vi "SubVI-AOMvolt-Power Calibration for 1064-v3.vi"() -> ()   [LabVIEW 2014]
uses:
  <vilib>/DAQmx/read.llb/DAQmx Read (Analog 1D DBL 1Chan NSamp).vi
  <vilib>/Analysis/NI_AALBase.lvlib
  <vilib>/Analysis/baseanly.llb/Mean (DBL).vi
  <vilib>/DAQmx/create/channels.llb/DAQmx Create Channel (AI-Voltage-Basic).vi
  <vilib>/DAQmx/configure/timing.llb/DAQmx Timing (Sample Clock).vi
  <vilib>/Utility/file.llb/Write To Spreadsheet File (DBL).vi
  <vilib>/Analysis/NI_AALPro.lvlib
  <vilib>/Analysis/polynomials.llb/Scalar Polynomial Evaluation (DBL).vi
panel:
  out "Raw data":T1
  in  "save cal curve?":bool
  out "Fit AOM volt(V)":dbl[](array[numeric])
  out "Fit laser power (mW)":dbl[](array[numeric])
  out "XY Graph":cluster{dbl[], dbl[]}[](graph)
  out "Polynomial Coefficients":dbl[](array[numeric]) format="%0.2f"
  in  "record z axis":bool
  in  "Physical Channel":tag="Dev1/ai4:5"
  in  "Samples per Channel":i32=1000
  in  "Rate":dbl=10000.0 caption="Sample Rate (Hz)" format="%0.2f"
  in  "Minimum Value":dbl=-10.0 format="%0.2f"
  in  "Maximum Value":dbl=10.0 format="%0.2f"
  in  "Set laser power (mW)":dbl=10.0 format="%#_13g"
  out "Choosed AOM volt":dbl
  out "Choosed laser power (mW)":dbl format="%#_13g"
  in  "warmup time (sec)":dbl=3.0
  in  "Min voltage":dbl=0.1
  out "powermeter readout (mW)":dbl
  out "power":dbl
  in  "instrument handle":refnum<visa-resource-name>
  in  "error in (no error)":errorcluster {"code" format="%.0x"}
  in  "milliseconds to wait":u32=300
  out "current voltage":dbl
  in  "Max voltage":dbl=5.0
  out "voltage step size":dbl=0.25
  in  "scan step #":dbl=20.0
  out "Voltage for AOM":dbl
  in  "stop":bool
  in  "Scanning cycles":dbl=1.0
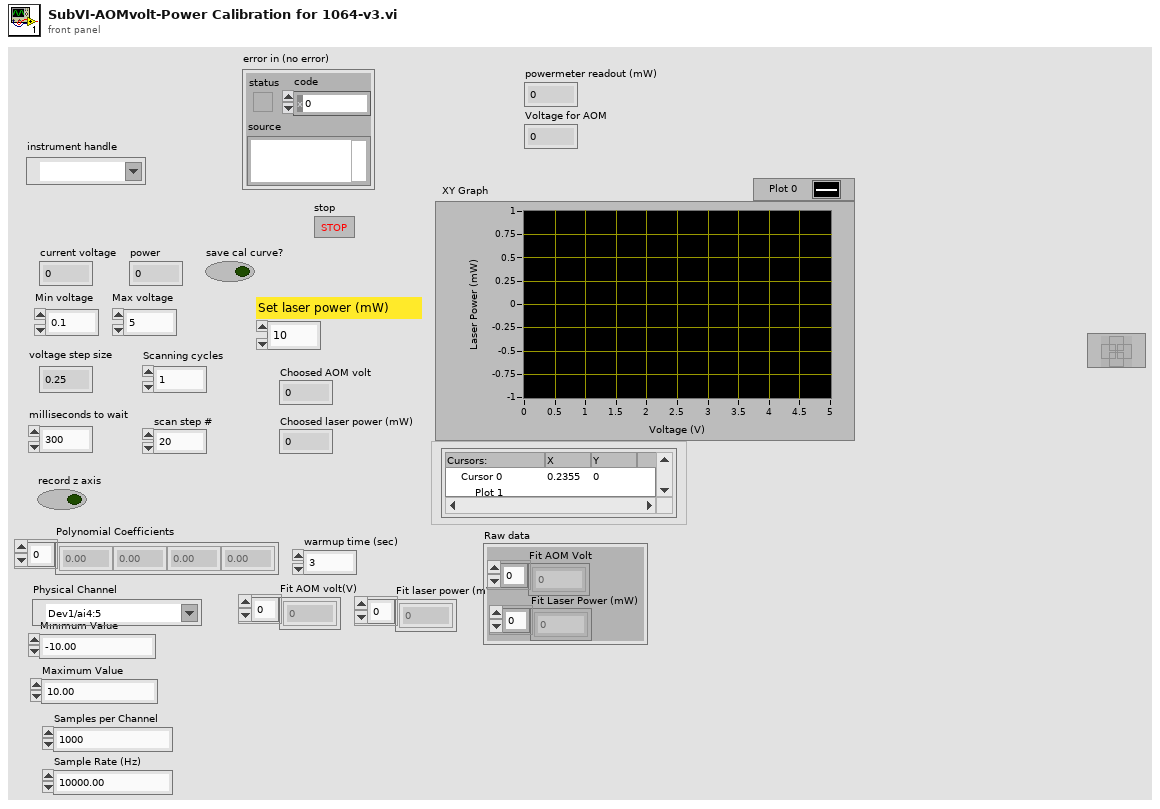
[diagram p1: front panel]
types:
  T1 = cluster{"Fit AOM Volt":dbl[], "Fit Laser Power (mW)":dbl[]}
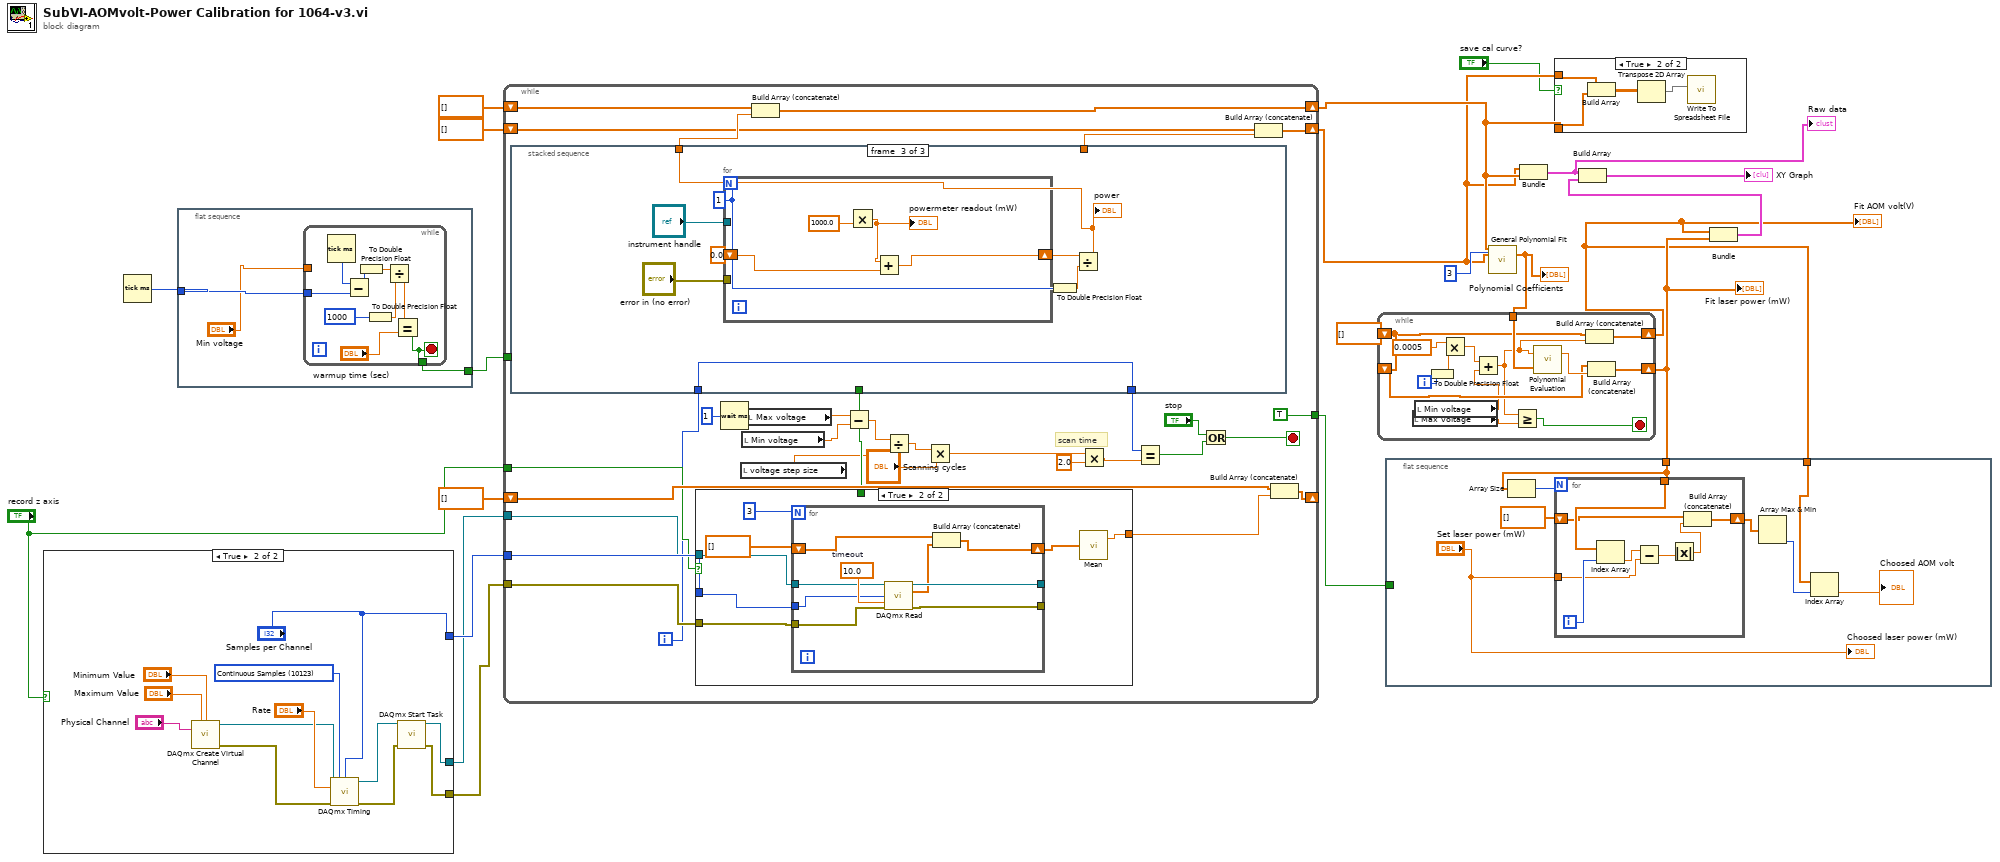
[diagram p0: block diagram]
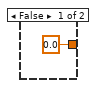
[diagram p4: hidden frame]
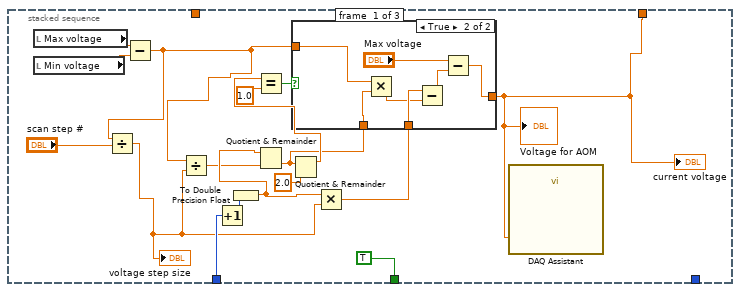
[diagram p5: hidden frame]
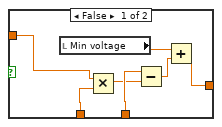
[diagram p6: hidden frame]
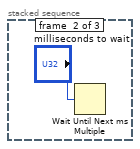
[diagram p7: hidden frame]
diagram:
  w11 = dbl[] []
  n1 = case shown="True" "record z axis" {
    tunnel: [_ "Samples per Channel"] -> w17
    tunnel: [_ w23] -> w16
    tunnel: [_ w22] -> w15
    frame False {
    }
    frame True {
      w28 = 10123 items=["Finite Samples"=10178, "Continuous Samples"=10123] ("sample mode")
      n2 = call-poly <vilib>:"DAQmx Create Virtual Channel.vi"("maximum value"="Maximum Value", "minimum value"="Minimum Value", "physical channels"="Physical Channel") -> ("task out"=w29:refnum<k21>, "error out"=w31:errorcluster)  [unwired: 6 in, 5 out]
      n3 = call-poly <vilib>:"DAQmx Timing.vi"("task/channels in"=w29, "sample mode"=w28, "samples per channel"="Samples per Channel", "rate"="Rate", "error in"=w31) -> ("task out"=w27:refnum<k21>, "error out"=w26:errorcluster)  [unwired: 2 in, 7 out]
      n4 = call <vilib>:"DAQmx Start Task.vi"("task/channels in"=w27, "error in"=w26) -> ("task out"=w23:refnum<k21>, "error out"=w22:errorcluster)  [unwired: 12 out]
    }
  }
  n5 = Tick Count (ms)() -> (millisecond timer value=w8:u32)
  n6 = flat-sequence {
    tunnel: w8 -> [w36]
    tunnel: [w35] -> w21
    frame #0 {
      n7 = while {
        tunnel: w36 -> [w44]
        tunnel: [w40] -> w35
        tunnel: "Min voltage" -> [_]
        stop <- w40 stop-if-true
        n8 = Tick Count (ms)() -> (millisecond timer value=w45:u32)
        n9 = Subtract(x=w45, y=w44) -> (x-y=w43:u32)
        n10 = To Double Precision Float(number=w43) -> (double precision float=w39:dbl)
        n11 = To Double Precision Float(number=u32 1000 ("y")) -> (double precision float=w38:dbl)
        n12 = Divide(x=w39, y=w38) -> (x/y=w41:dbl)
        n13 = Equal?(x=w41, y="warmup time (sec)") -> (x = y?=w40:bool)
      }
    }
  }
  n14 = while {
    tunnel: w21 -> [_]
    shift-right: [w73] -> w7
    shift-left: dbl[] [] -> [w70]
    shift-right: [w74] -> w6
    shift-left: dbl[] [] -> [w69]
    tunnel: [TRUE] -> w18
    tunnel: w17 -> [w67]
    tunnel: w16 -> [w66]
    tunnel: w15 -> [w65]
    shift-right: [w63] -> _
    shift-left: dbl[] [] -> [w62]
    tunnel: "record z axis" -> [w61]
    i -> [w59]
    stop <- w57 stop-if-true
    # "scan time"
    n15 = stacked-sequence {
      tunnel: [w93 _ _] -> w72
      tunnel: [_ _ w128] -> w71
      tunnel: [TRUE _ _] -> w60
      tunnel: w59 -> [w101 _ w131]
      tunnel: [_ _ w131] -> w56
      frame #0 {
        n16 = local read "Max voltage"() -> (w99:dbl)
        n17 = local read "Min voltage"() -> (w98:dbl)
        n18 = Subtract(x=w99, y=w98) -> (x-y=w96:dbl)
        n19 = Divide(x=w96, y="scan step #") -> (x/y=w94:dbl)
        "voltage step size" <- w94
        n20 = Divide(x=w96, y=w94) -> (x/y=w97:dbl)
        n21 = Increment(x=w101) -> (x+1=w108:i32)
        n22 = To Double Precision Float(number=w108) -> (double precision float=w100:dbl)
        n23 = Quotient & Remainder(x=w100, y=w97) -> (floor(x/y)=w102:dbl)  [unwired: 1 out]
        n24 = Quotient & Remainder(x=w102, y=2.0) -> (x-y*floor(x/y)=w104:dbl)  [unwired: 1 out]
        n25 = Equal?(x=w104, y=1.0) -> (x = y?=w105:bool)
        n26 = Multiply(x=w100, y=w94) -> (x*y=w107:dbl)
        n27 = case shown="True" w105 {
          tunnel: w107 -> [w114 w122]
          tunnel: [w116 w123] -> w93
          tunnel: w102 -> [w115 w119]
          tunnel: w96 -> [w111 w117]
          frame False {
            n28 = local read "Min voltage"() -> (w110:dbl)
            n29 = Multiply(x=w111, y=w115) -> (x*y=w113:dbl)
            n30 = Subtract(x=w114, y=w113) -> (x-y=w112:dbl)
            n31 = Add(x=w110, y=w112) -> (x+y=w116:dbl)
          }
          frame True {
            n32 = Multiply(x=w117, y=w119) -> (x*y=w121:dbl)
            n33 = Subtract(x=w122, y=w121) -> (x-y=w120:dbl)
            n34 = Subtract(x="Max voltage", y=w120) -> (x-y=w123:dbl)
          }
        }
        "current voltage" <- w93
        "Voltage for AOM" <- w93
        n35 = call "DAQ Assistant"("data"=w93) -> ()  [unwired: 17 in, 2 out]
      }
      frame #1 {
        n36 = Wait Until Next ms Multiple(millisecond multiple="milliseconds to wait") -> ()  [unwired: 1 out]
      }
      frame #2 {
        w129 = 1
        n37 = for {
          N: w129 -> [_]
          shift-right: [w136] -> w130
          shift-left: 0.0 -> [w135]
          tunnel: "instrument handle" -> [_]
          tunnel: "error in (no error)" -> [_]
          n38 = Multiply(y=1000.0) -> (x*y=w133:dbl)  [unwired: 1 in]
          "powermeter readout (mW)" <- w133
          n39 = Add(x=w133, y=w135) -> (x+y=w136:dbl)
        }
        n40 = To Double Precision Float(number=w129) -> (double precision float=w127:dbl)
        n41 = Divide(x=w130, y=w127) -> (x/y=w128:dbl)
        "power" <- w128
      }
    }
    n42 = case shown="True" w61 {
      tunnel: w67 -> [_ w83]
      tunnel: w66 -> [_ w82]
      tunnel: w65 -> [_ w81]
      tunnel: [0.0 ("mean") w80] -> w64
      tunnel: w60 -> [_ _]
      frame False {
      }
      frame True {
        n43 = for {
          N: 3 -> [_]
          tunnel: [w92] -> _
          tunnel: [w91] -> _
          shift-right: [w84] -> w77
          shift-left: dbl[] [] -> [w90]
          tunnel: w82 -> [w87]
          tunnel: w83 -> [w86]
          tunnel: w81 -> [w85]
          w89 = 10.0  # timeout
          n44 = call-poly <vilib>:"DAQmx Read.vi"("task/channels in"=w87, "number of samples per channel"=w86, "timeout"=w89, "error in"=w85) -> ("task out"=w92:refnum<k21>, "data"=w88:dbl[], "error out"=w91:errorcluster)  [unwired: 9 out]
          n45 = Build Array (concatenate) "Build Array"(w90, w88) -> (w84:dbl[])
        }
        n46 = call-poly <vilib>:"Mean.vi"("X"=w77) -> ("mean"=w80:dbl)  [unwired: 1 out]
      }
    }
    n47 = Wait (ms)(milliseconds to wait=u32 1) -> ()  [unwired: 1 out]
    n48 = local read "voltage step size"() -> (w51:dbl)
    n49 = local read "Min voltage"() -> (w53:dbl)
    n50 = local read "Max voltage"() -> (w54:dbl)
    n51 = Build Array (concatenate)(w70, w71) -> (w73:dbl[])
    n52 = Subtract(x=w54, y=w53) -> (x-y=w52:dbl)
    n53 = Divide(x=w52, y=w51) -> (x/y=w50:dbl)
    n54 = Multiply(x=w50, y="Scanning cycles") -> (x*y=w47:dbl)
    n55 = Multiply(x=w47, y=2.0) -> (x*y=w48:dbl)
    n56 = Equal?(x=w56, y=w48) -> (x = y?=w55:bool)
    n57 = Or(x="stop", y=w55) -> (x .or. y?=w57:bool)
    n58 = Build Array (concatenate)(w69, w72) -> (w74:dbl[])
    n59 = Build Array (concatenate)(w62, w64) -> (w63:dbl[])
  }
  n60 = flat-sequence {
    tunnel: w18 -> [_]
    tunnel: w3 -> [w138]
    tunnel: w2 -> [w141]
    frame #0 {
      n61 = Array Size(array=w138) -> (size(s)=w137:i32)
      n62 = for {
        N: w137 -> [_]
        tunnel: w138 -> [w152]
        tunnel: "Set laser power (mW)" -> [w149]
        shift-right: [w146] -> w142
        shift-left: dbl[] [] -> [w145]
        i -> [w151]
        n63 = Index Array(array=w152, index=w151) -> (element=w150:dbl)
        n64 = Subtract(x=w150, y=w149) -> (x-y=w148:dbl)
        n65 = Absolute Value(x=w148) -> (abs(x)=w147:dbl)
        n66 = Build Array (concatenate)(w145, w147) -> (w146:dbl[])
      }
      n67 = Array Max & Min(array=w142) -> (min index (indices)=w140:i32)  [unwired: 3 out]
      n68 = Index Array(array=w141, index=w140) -> (element=→"Choosed AOM volt":dbl)
      "Choosed laser power (mW)" <- "Set laser power (mW)"
    }
  }
  n69 = call <vilib>:"General Polynomial Fit.vi"("Y"=w7, "polynomial order"=3, "X"=w6) -> ("Polynomial Coefficients"=w4:dbl[])  [unwired: 9 in, 3 out]
  "Polynomial Coefficients" <- w4
  n70 = while {
    tunnel: w4 -> [w162]
    shift-right: [w161] -> w2
    shift-left: w11 -> [w158]
    shift-right: [w159] -> w3
    shift-left: w11 -> [w157]
    i -> [w166]
    stop <- w155 stop-if-true
    n71 = local read "Max voltage"() -> (w154:dbl)
    n72 = local read "Min voltage"() -> (w153:dbl)
    n73 = To Double Precision Float(number=w166) -> (double precision float=w165:dbl)
    n74 = Multiply(x=0.0005, y=w165) -> (x*y=w163:dbl)
    n75 = Add(x=w163, y=w153) -> (x+y=w156:dbl)
    n76 = Greater Or Equal?(x=w156, y=w154) -> (x >= y?=w155:bool)
    n77 = call-poly <vilib>:"Polynomial Evaluation.vi"("P(x)"=w162, "a"=w156) -> ("P(a)"=w160:dbl)  [unwired: 1 out]
    n78 = Build Array (concatenate)(w158, w156) -> (w161:dbl[])
    n79 = Build Array (concatenate)(w157, w160) -> (w159:dbl[])
  }
  "Fit laser power (mW)" <- w3
  "Fit AOM volt(V)" <- w2
  n80 = Bundle(w6, w7) -> (w1:cluster{dbl[], dbl[]})  [unwired: 1 out]
  "Raw data" <- w1
  n81 = case shown="True" "save cal curve?" {
    tunnel: w7 -> [_ w170]
    tunnel: w6 -> [_ w169]
    frame False {
    }
    frame True {
      n82 = Build Array(w169, w170) -> (w168:dbl[][])
      n83 = Transpose 2D Array(2D array=w168) -> (transposed array=w167:dbl[][])
      n84 = call-poly <vilib>:"Write To Spreadsheet File.vi"("2D data"=w167) -> ()  [unwired: 5 in, 3 out]
    }
  }
  n85 = Bundle(w2, w3) -> (w10:cluster{dbl[], dbl[]})  [unwired: 1 out]
  n86 = Build Array(w1, w10) -> (→"XY Graph":cluster{dbl[], dbl[]}[])
